vi "Shifting.vi"(10 "Downshift RPM":dbl, 11 "Upshift RPM":dbl) -> ()   [LabVIEW 2015]
uses:
  <vilib>/Rock Robotics/WPI/Solenoid/WPI_SolenoidValue.ctl
  Robot Global Data.vi
  <vilib>/Rock Robotics/WPI/Solenoid/WPI_SolenoidSetEnum.vi
panel:
  out "Auto Shift?":bool
  in  "Test Mode":bool
  in  "Motor RPM":dbl(slide) scale=0.0..10000.0
  out "Gear":bool
  # "If test mode, motor ignores actual RPM\nand outputs this simulated one"
  # "ON=Auto\nOFF=Man"
  # "ON=High\nOFF=Low"
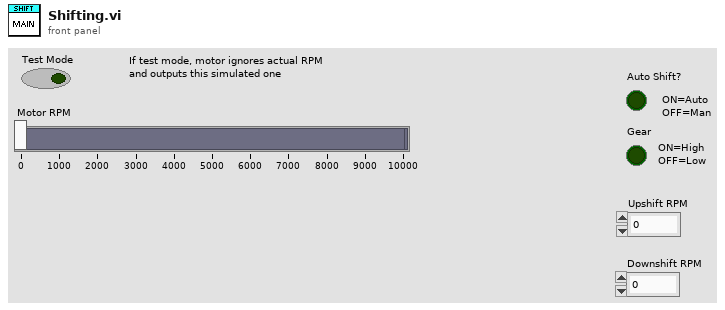
[diagram p1: front panel]
types:
  T1 = typedef "WPI_SolenoidDevRef.ctl" = cluster{"DevStatus":errorcluster, "Pneumatics Control Module":u8, "Forward Solenoid Channel":T2, "Reverse Solenoid Channel":T2}
  T2 = typedef "WPI_SolenoidChannel.ctl" = enum8{"Solenoid 0", "Solenoid 1", "Solenoid 2", "Solenoid 3", "Solenoid 4", "Solenoid 5", "Solenoid 6", "Solenoid 7", "Invalid"}
  T3 = typedef "WPI_EncoderDevRef.ctl" = cluster{"DevStatus":errorcluster, "EncoderIndex":T4, "CounterIndex":T5, "DistancePerCount":dbl, "Decoding Type":T6}
  T4 = typedef "FPGA_EncoderIdx.ctl" = enum8{"Enc 0", "Enc 1", "Enc 2", "Enc 3", "Enc 4", "Enc 5", "Enc 6", "Enc 7", "Invalid"}
  T5 = typedef "FPGA_CounterCtrSystemIndex.ctl" = enum8{"Ctr 0", "Ctr 1", "Ctr 2", "Ctr 3", "Ctr 4", "Ctr 5", "Ctr 6", "Ctr 7", "Invalid"}
  T6 = typedef "WPI_EncoderType.ctl" = enum16{"1x", "2x", "4x"}
  T7 = typedef "WPI_SolenoidValue.ctl" = enum16{"Off", "On", "Forward", "Reverse"}
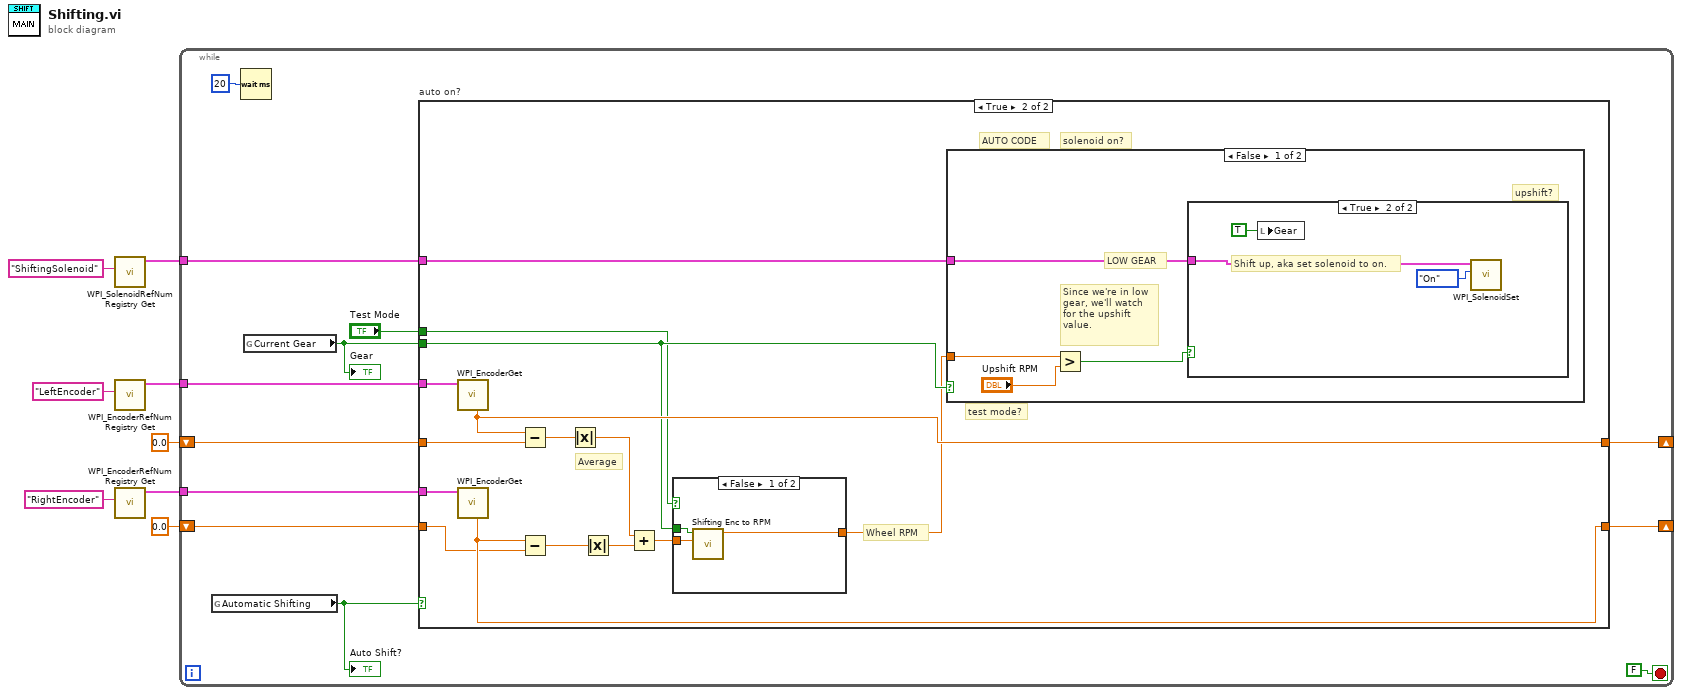
[diagram p0: block diagram]
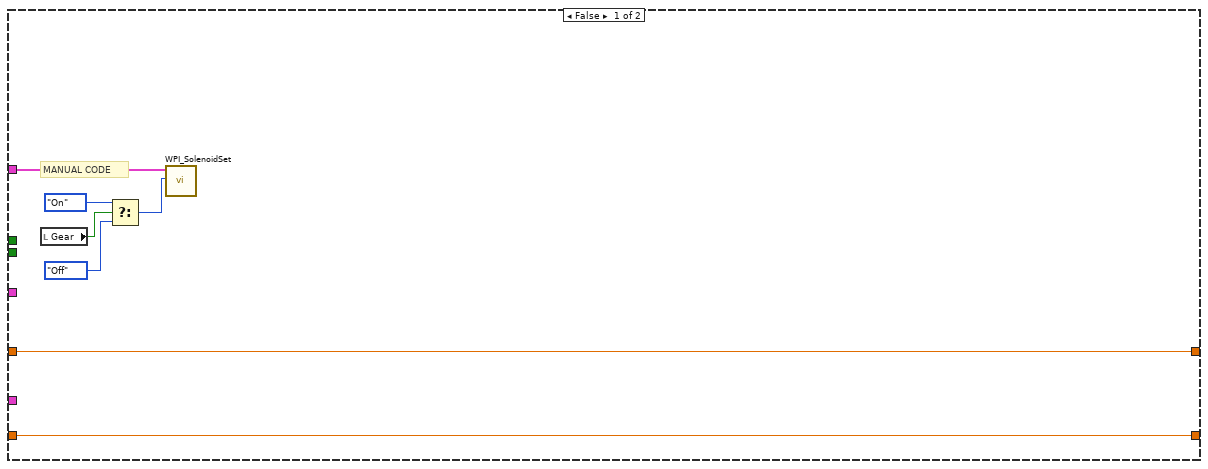
[diagram p2: hidden frame]
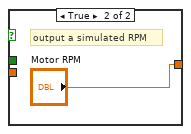
[diagram p3: hidden frame]
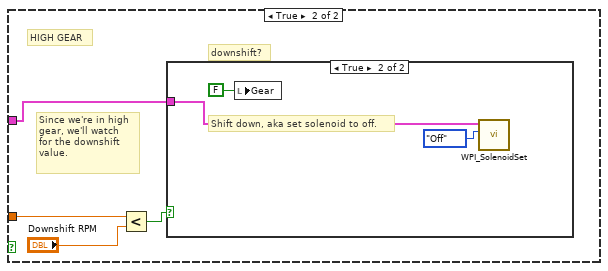
[diagram p5: hidden frame]
diagram:
  n1 = call <vilib>:"WPI_SolenoidRefNum Registry Get.vi"("refnum name"="ShiftingSolenoid") -> ("SolenoidDevRef"=w3:T1)  [unwired: 9 in, 1 out]
  n2 = call <vilib>:"WPI_EncoderRefNum Registry Get.vi"("refnum name"="LeftEncoder") -> ("EncoderDevRef"=w5:T3)  [unwired: 9 in, 1 out]
  n3 = call <vilib>:"WPI_EncoderRefNum Registry Get.vi"("refnum name"="RightEncoder") -> ("EncoderDevRef"=w4:T3)  [unwired: 9 in, 1 out]
  n4 = while {
    tunnel: w5 -> [w19]
    tunnel: w4 -> [w18]
    shift-right: [w17] -> _
    shift-left: 0.0 ("Rate") -> [w15]
    shift-right: [w16] -> _
    shift-left: 0.0 ("Rate") -> [w14]
    tunnel: w3 -> [w11]
    stop <- FALSE stop-if-true
    n5 = global read "Robot Global Data.vi" "Automatic Shifting"() -> (w10:bool)
    "Auto Shift?" <- w10
    n6 = Wait (ms)(milliseconds to wait=u32 20) -> ()  [unwired: 1 out]
    n7 = global read "Robot Global Data.vi" "Current Gear"() -> (w9:bool)
    "Gear" <- w9
    n8 = case "auto on?" shown="True" w10 {
      tunnel: w11 -> [w21 w30]
      tunnel: w19 -> [_ w42]
      tunnel: w18 -> [_ w41]
      tunnel: [w27 w40] -> w17
      tunnel: [w26 w38] -> w16
      tunnel: w15 -> [w27 w39]
      tunnel: w14 -> [w26 w37]
      tunnel: w9 -> [_ w31]
      tunnel: "Test Mode" -> [_ w28]
      frame False {
        # "MANUAL CODE"
        n9 = local read "Gear"() -> (w22:bool)
        n10 = Select(t=WPI_SolenoidValue."On", s=w22, f=WPI_SolenoidValue."Off" ("Value")) -> (s? t:f=w25:T7)
        n11 = call-poly <vilib>:"WPI_SolenoidSet.vi"("Value"=w25, "SolenoidDevRef"=w21) -> ()  [unwired: 8 in, 2 out]
      }
      frame True {
        # "Average"
        # "test mode?"
        # "solenoid on?"
        # "Wheel RPM"
        # "AUTO CODE"
        n12 = call <vilib>:"WPI_EncoderGet.vi"("EncoderDevRef"=w42) -> ("Rate"=w40:dbl)  [unwired: 5 in, 5 out]
        n13 = call <vilib>:"WPI_EncoderGet.vi"("EncoderDevRef"=w41) -> ("Rate"=w38:dbl)  [unwired: 5 in, 5 out]
        n14 = Subtract(x=w40, y=w39) -> (x-y=w36:dbl)
        n15 = Subtract(x=w38, y=w37) -> (x-y=w35:dbl)
        n16 = Absolute Value(x=w36) -> (abs(x)=w34:dbl)
        n17 = Absolute Value(x=w35) -> (abs(x)=w33:dbl)
        n18 = Add(x=w34, y=w33) -> (x+y=w32:dbl)
        n19 = case shown="False" w28 {
          tunnel: w32 -> [w45 _]
          tunnel: w31 -> [w44 _]
          tunnel: [w43 "Motor RPM"] -> w29
          frame False {
            n20 = call "Shifting Enc to RPM.vi"("Encoder Value"=w45, "Current Gear"=w44) -> ("RPM"=w43:dbl)  [unwired: 9 in]
          }
          frame True {
            # "output a simulated RPM"
          }
        }
        n21 = case shown="False" w31 {
          tunnel: w29 -> [w50 w54]
          tunnel: w30 -> [w47 w55]
          frame False {
            # "Since we're in low\ngear, we'll watch\nfor the upshift\nvalue."
            # "LOW GEAR"
            # "upshift?"
            n22 = Greater?(x=w50, y="Upshift RPM") -> (0:w48:bool)
            n23 = case shown="True" w48 {
              tunnel: w47 -> [_ w53]
              frame False {
                # "Since we don't need to upshift, we don't do anything."
              }
              frame True {
                # "Shift up, aka set solenoid to on."
                n24 = local write "Gear"(TRUE) -> ()
                n25 = call-poly <vilib>:"WPI_SolenoidSet.vi"("Value"=WPI_SolenoidValue."On", "SolenoidDevRef"=w53) -> ()  [unwired: 8 in, 2 out]
              }
            }
          }
          frame True {
            # "HIGH GEAR"
            # "Since we're in high\ngear, we'll watch\nfor the downshift\nvalue."
            # "downshift?"
            n26 = Less?(x=w54, y="Downshift RPM") -> (x < y?=w57:bool)
            n27 = case shown="True" w57 {
              tunnel: w55 -> [_ w60]
              frame False {
                # "Since we don't need to downshift, we don't do anything."
              }
              frame True {
                # "Shift down, aka set solenoid to off."
                n28 = local write "Gear"(FALSE) -> ()
                n29 = call-poly <vilib>:"WPI_SolenoidSet.vi"("Value"=WPI_SolenoidValue."Off", "SolenoidDevRef"=w60) -> ()  [unwired: 8 in, 2 out]
              }
            }
          }
        }
      }
    }
  }
